vi "create.vi"(8 "error in (no error)":errorcluster, 10 "configuration":T1, 11 "console.provider in":refnum<class "console.provider.lvclass">) -> (0 "error out":errorcluster, 3 "console.provider out":refnum<class "console.provider.lvclass">)   [LabVIEW 2021, in "console.provider.lvclass"]
uses:
  console.provider.lvclass
  system.logging/configuration.ctl
  console_payload.ctl
  console_commands.ctl
  system.logging/log_entry.ctl
  system.logging/severity.ctl
  console.provider.lvclass/console.provider.ctl
  system.logging.provider.lvclass
  system.logging/system.logging.lvclass
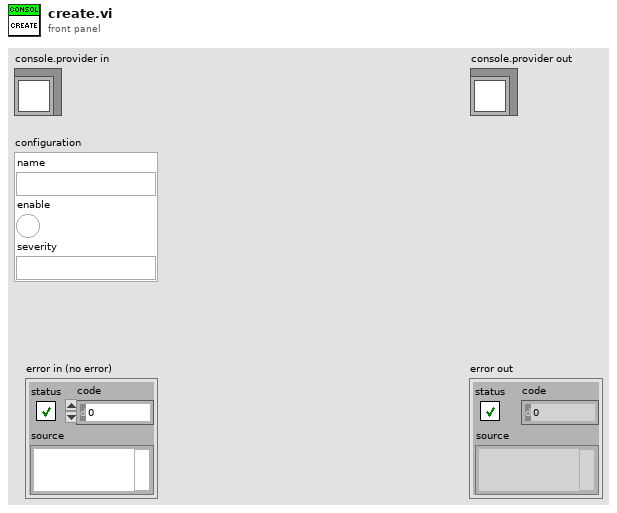
[diagram p1: front panel]
types:
  T1 = typedef "system.logging.lvclass/configuration.ctl" = cluster{"name":string, "enable":bool, "severity":string}
  T2 = typedef "console.provider.lvclass/console_payload.ctl" = cluster{"console_cmd":T3, "log":T4}
  T3 = typedef "console.provider.lvclass/console_commands.ctl" = enum16{"close", "print"}
  T4 = typedef "system.logging.lvclass/log_entry.ctl" = cluster{"severity":T5, "message":string, "origin":string, "datetime":timestamp}
  T5 = typedef "system.logging.lvclass/severity.ctl" = enum8{"trace", "debug", "info", "warning", "error"}
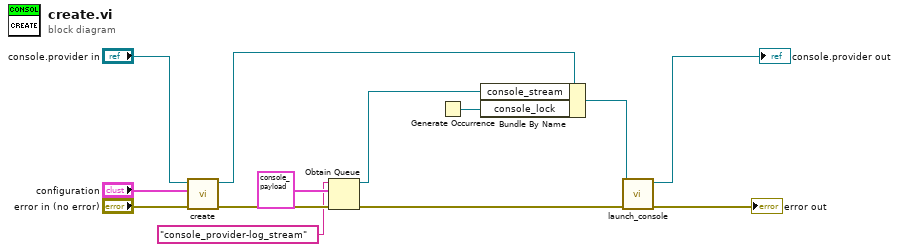
[diagram p0: block diagram]
diagram:
  n1 = call-parent "create.vi"("error in (no error)"="error in (no error)", "configuration"="configuration", "system.logging.provider in"="console.provider in") -> ("error out"=w9:errorcluster, "system.logging.provider out"=w10:refnum<class "console.provider.lvclass">)  [unwired: 7 in]
  n2 = Obtain Queue(name (unnamed)="console_provider-log_stream", element data type=T2 {"console_cmd"=enum."close", "log"={"severity"=enum."trace", "message"="", "origin"="", "datetime"=timestamp(0 s since 1904-01-01)}} ("console_payload"), error in (no error)=w9) -> (queue out=w3:refnum<queue>, error out=w7:errorcluster)  [unwired: 2 in, 1 out]
  n3 = Generate Occurrence() -> (w1:refnum<k4>)
  n4 = Bundle By Name(cluster=w10, "console_stream"=w3, "console_lock"=w1) -> (w6:refnum<class "console.provider.lvclass">)
  n5 = call "launch_console.vi"("error (in)"=w7, "console.provider.lvclass"=w6) -> ("error (out)"=→"error out":errorcluster, "console.provider (out)"=→"console.provider out":refnum<class "console.provider.lvclass">)  [unwired: 8 in]
